vi "HW4p1_bartelmj.vi"() -> ()   [LabVIEW 2016]
uses:
  <vilib>/express/express arith-compare/Formula/XNode/ExpressFormulaBlockNode.xnode
panel:
  out "displacment (p)":dbl
  out "potential energy (PE)":dbl
  out "acceleration (a)":dbl
  out "velocity (v)":dbl
  out "Kenetic energy (Ke)":dbl
  in  "Time (t)":dbl
  in  "Mass of object (m)":dbl
  in  "spring constant (k)":dbl
  in  "initial displacment (a)":dbl
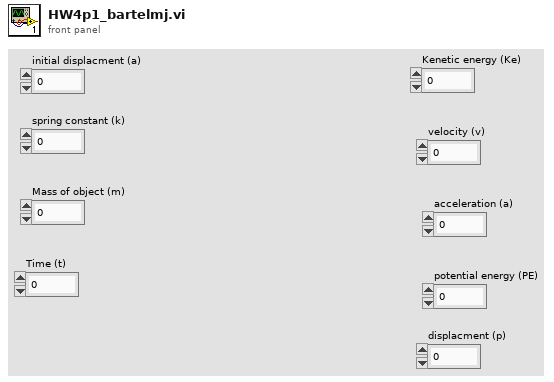
[diagram p1: front panel]
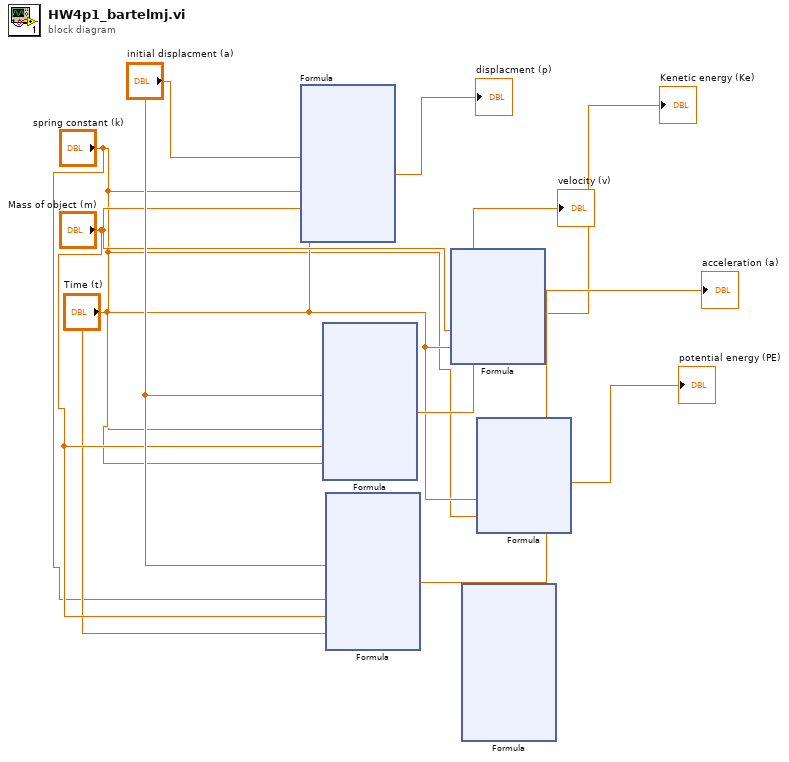
[diagram p0: block diagram]
diagram:
  n1 = xnode "Formula"("A"="initial displacment (a)", "k"="spring constant (k)", "m"="Mass of object (m)", "t"="Time (t)") -> ("Result"=→"displacment (p)":dbl)  [unwired: 1 in, 1 out]
  n2 = xnode "Formula"("A"="initial displacment (a)", "k"="spring constant (k)", "m"="Mass of object (m)", "t"="Time (t)") -> ("Result"=→"velocity (v)":dbl)  [unwired: 1 in, 1 out]
  n3 = xnode "Formula"("A"="initial displacment (a)", "k"="spring constant (k)", "m"="Mass of object (m)", "t"="Time (t)") -> ("Result"=→"acceleration (a)":dbl)  [unwired: 1 in, 1 out]
  n4 = xnode "Formula"("m"="Mass of object (m)", "t"="Time (t)") -> ("Result"=→"Kenetic energy (Ke)":dbl)  [unwired: 1 in, 1 out]
  n5 = xnode "Formula"() -> ()  [unwired: 5 in, 2 out]
  n6 = xnode "Formula"("t"="Time (t)", "k"="spring constant (k)") -> ("Result"=→"potential energy (PE)":dbl)  [unwired: 1 in, 1 out]
